vi "Test RoundTrip Enumeration.vi"(8 "error in (no error)":errorcluster) -> (0 "error out":errorcluster)   [LabVIEW 2013]
uses:
  <vilib>/addons/_JKI Toolkits/Caraya/classes/Test/Test.lvclass
  <vilib>/addons/_JKI Toolkits/Caraya/classes/Assert/Assert.lvclass
  src/JKI JSON Serialization.lvlib
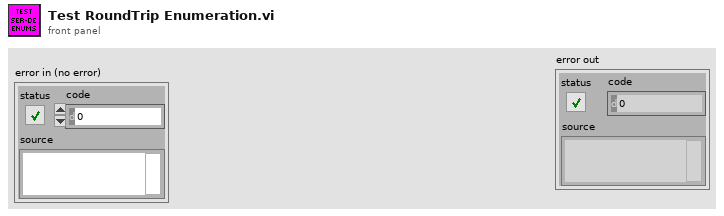
[diagram p1: front panel]
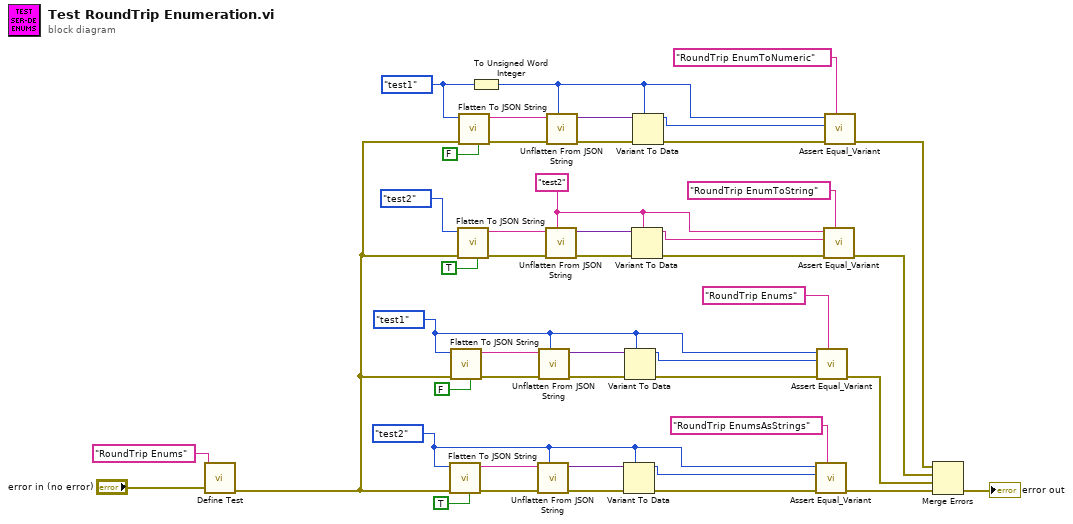
[diagram p0: block diagram]
diagram:
  w3 = "test2" ("Label (VI Title)")
  w5 = enum16{"test", "test1", "test2"}."test1"
  w33 = enum16{"test", "test1", "test2"}."test1"
  w34 = enum16{"test", "test1", "test2"}."test2"
  n1 = call <vilib>:"Define Test.vi"("error in (no error)"="error in (no error)", "Label (VI Title)"="RoundTrip Enums") -> ("error out"=w6:errorcluster)  [unwired: 9 in]
  n2 = call "Flatten To JSON String.vi"("Enums As String (F)"=TRUE, "error in (no error)"=w6, "Variant"=w34) -> ("error out"=w41:errorcluster, "JSON String"=w40:string)  [unwired: 7 in]
  n3 = call "Flatten To JSON String.vi"("Enums As String (F)"=FALSE, "error in (no error)"=w6, "Variant"=w33) -> ("error out"=w26:errorcluster, "JSON String"=w27:string)  [unwired: 7 in]
  n4 = call "Flatten To JSON String.vi"("Enums As String (F)"=TRUE, "error in (no error)"=w6, "Variant"=enum16{"test", "test1", "test2"}."test2") -> ("error out"=w8:errorcluster, "JSON String"=w9:string)  [unwired: 7 in]
  n5 = call "Flatten To JSON String.vi"("Enums As String (F)"=FALSE, "error in (no error)"=w6, "Variant"=w5) -> ("error out"=w22:errorcluster, "JSON String"=w21:string)  [unwired: 7 in]
  n6 = To Unsigned Word Integer(number=w5) -> (unsigned 16bit integer=w4:u16)
  n7 = call "Unflatten From JSON String.vi"("Type and Defaults"=w34, "error in (no error)"=w41, "JSON String"=w40) -> ("error out"=w36:errorcluster, "Variant"=w38:variant)  [unwired: 7 in]
  n8 = call "Unflatten From JSON String.vi"("Type and Defaults"=w33, "error in (no error)"=w26, "JSON String"=w27) -> ("error out"=w31:errorcluster, "Variant"=w29:variant)  [unwired: 7 in]
  n9 = call "Unflatten From JSON String.vi"("Type and Defaults"=w3, "error in (no error)"=w8, "JSON String"=w9) -> ("error out"=w13:errorcluster, "Variant"=w11:variant)  [unwired: 7 in]
  n10 = call "Unflatten From JSON String.vi"("Type and Defaults"=w4, "error in (no error)"=w22, "JSON String"=w21) -> ("error out"=w17:errorcluster, "Variant"=w19:variant)  [unwired: 7 in]
  n11 = Variant To Data(error in=w36, type=w34, Variant=w38) -> (data=w37:enum16{"test", "test1", "test2"}, error out=w35:errorcluster)
  n12 = Variant To Data(error in=w31, type=w33, Variant=w29) -> (data=w30:enum16{"test", "test1", "test2"}, error out=w32:errorcluster)
  n13 = Variant To Data(error in=w13, type=w3, Variant=w11) -> (data=w12:string, error out=w14:errorcluster)
  n14 = Variant To Data(error in=w17, type=w4, Variant=w19) -> (data=w18:u16, error out=w16:errorcluster)
  n15 = call <vilib>:"Assert Equal_Variant.vi"("Label"="RoundTrip EnumsAsStrings", "error in (no error)"=w35, "Y"=w37, "X"=w34) -> ("error out"=w43:errorcluster)  [unwired: 7 in]
  n16 = call <vilib>:"Assert Equal_Variant.vi"("Label"="RoundTrip Enums", "error in (no error)"=w32, "Y"=w30, "X"=w33) -> ("error out"=w24:errorcluster)  [unwired: 7 in]
  n17 = call <vilib>:"Assert Equal_Variant.vi"("Label"="RoundTrip EnumToString", "error in (no error)"=w14, "Y"=w12, "X"=w3) -> ("error out"=w2:errorcluster)  [unwired: 7 in]
  n18 = call <vilib>:"Assert Equal_Variant.vi"("Label"="RoundTrip EnumToNumeric", "error in (no error)"=w16, "Y"=w18, "X"=w4) -> ("error out"=w1:errorcluster)  [unwired: 7 in]
  n19 = Merge Errors(w1, w2, w24, w43) -> (→"error out":errorcluster)
